vi "PH_Tektronix_7000.Evt Call Set Acquisition Configuration.vi"(0 "i ref in":refnum<vi>, 1 "Instance":string="N/A", 2 "Acquisition Configuration":T1={"Record Length"=0, "Timebase [s/div]"=10000.0, "Position [%]"=0.0, "Acquisition Type"=1, "Average Waveforms"=10, "Envelope Waveforms"=10, "WfmDB Samples"=16000, "Continuous?"=FALSE, "Delay [s]"=0.0, "Run?"=FALSE} {"Delay [s]" format="%#_12p"; "Acquisition Type" items=["Sample", "Peak Detect", "Hi Res", "Average", "Envelope", "WfmDB"]; "Timebase [s/div]" format="%#_12g"}, 5 "error in (no error)":errorcluster) -> (14 "i ref out":refnum<vi>, 19 "error out":errorcluster)   [LabVIEW 2014, in "PH_Tektronix_7000.lvlib"]
doc: "This VI calls sets a simple call."
uses:
  PH_Tektronix_7000.lvlib
  PH_Tektronix_7000.Acquisition Config.ctl
  CSCore/CSSystem/CoreLib/CoreLib.int 2 byte array.vi
  CSCore/CSSystem/CoreLib/CoreLib.double 2 byte array.vi
  CSCore/CSSystem/CoreLib/CoreLib.short 2 byte array.vi
  CSCore/CSSystem/CoreLib/CoreLib.lvlib
  CSCore/BaseProcess/BaseProcess.lvlib
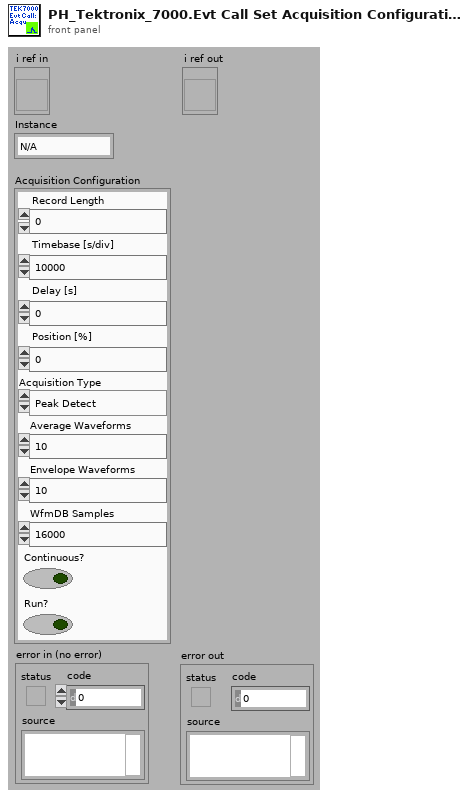
[diagram p1: front panel]
types:
  T1 = typedef "PH_Tektronix_7000.lvlib/PH_Tektronix_7000.Acquisition Config.ctl" = cluster{"Record Length":u32, "Timebase [s/div]":dbl, "Position [%]":dbl, "Acquisition Type":u16, "Average Waveforms":i32, "Envelope Waveforms":i32, "WfmDB Samples":i32, "Continuous?":bool, "Delay [s]":dbl, "Run?":bool}
  T2 = typedef "CoreDefs.rawDataType.ctl" = i8[]
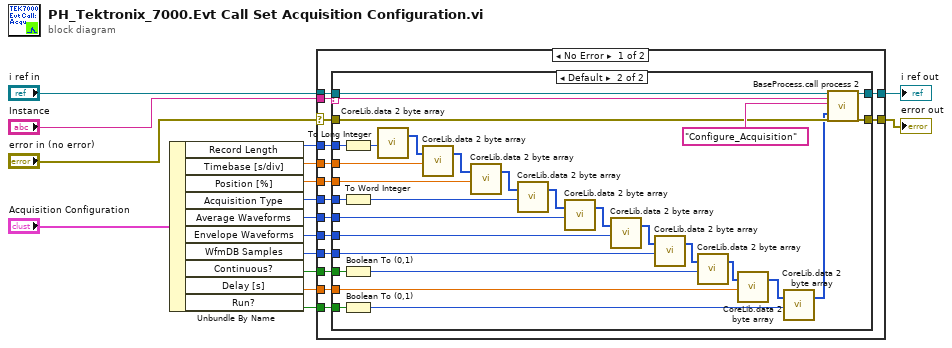
[diagram p0: block diagram]
diagram:
  n1 = Unbundle By Name("Acquisition Configuration") -> ("Record Length"=w10:u32, "Timebase [s/div]"=w9:dbl, "Position [%]"=w8:dbl, "Acquisition Type"=w7:u16, "Average Waveforms"=w6:i32, "Envelope Waveforms"=w4:i32, "WfmDB Samples"=w3:i32, "Continuous?"=w5:bool, "Delay [s]"=w2:dbl, "Run?"=w1:bool)
  n2 = case shown="No Error" "error in (no error)" {
    selector: "error in (no error)" -> [w27 w64]
    tunnel: [w31 w65] -> w16
    tunnel: [w30 w64] -> w15
    tunnel: "i ref in" -> [w29 w65]
    tunnel: w10 -> [w26 _]
    tunnel: "Instance" -> [w28 _]
    tunnel: w9 -> [w25 _]
    tunnel: w8 -> [w24 _]
    tunnel: w7 -> [w23 _]
    tunnel: w6 -> [w22 _]
    tunnel: w5 -> [w21 _]
    tunnel: w4 -> [w20 _]
    tunnel: w3 -> [w19 _]
    tunnel: w2 -> [w18 _]
    tunnel: w1 -> [w17 _]
    frame No Error {
      n3 = case shown="Default" w28 {
        selector: w28 -> [_ w58]
        tunnel: [w32 w62] -> w31
        tunnel: [w33 w61] -> w30
        tunnel: w29 -> [w32 w60]
        tunnel: w27 -> [w33 w59]
        tunnel: w26 -> [_ w57]
        tunnel: w25 -> [_ w48]
        tunnel: w24 -> [_ w55]
        tunnel: w23 -> [_ w53]
        tunnel: w22 -> [_ w46]
        tunnel: w21 -> [_ w50]
        tunnel: w20 -> [_ w44]
        tunnel: w19 -> [_ w42]
        tunnel: w18 -> [_ w39]
        tunnel: w17 -> [_ w38]
        frame "N/A" {
        }
        frame Default {
          n4 = To Long Integer(number=w57) -> (32bit integer=w49:i32)
          n5 = To Word Integer(number=w53) -> (16bit integer=w47:i16)
          n6 = Boolean To (0,1)(Boolean=w50) -> (0, 1=w52:i16)
          n7 = Boolean To (0,1)(Boolean=w38) -> (0, 1=w37:i16)
          n8 = call-poly "CoreLib.data 2 byte array.vi"("i32"=w49) -> ("byteArray out"=w56:T2)  [unwired: 18 in]
          n9 = call-poly "CoreLib.data 2 byte array.vi"("byteArray"=w56, "f64"=w48) -> ("byteArray out"=w54:T2)  [unwired: 17 in]
          n10 = call-poly "CoreLib.data 2 byte array.vi"("byteArray"=w54, "f64"=w55) -> ("byteArray out"=w51:T2)  [unwired: 17 in]
          n11 = call-poly "CoreLib.data 2 byte array.vi"("byteArray"=w51, "i16"=w47) -> ("byteArray out"=w45:T2)  [unwired: 17 in]
          n12 = call-poly "CoreLib.data 2 byte array.vi"("byteArray"=w45, "i32"=w46) -> ("byteArray out"=w43:T2)  [unwired: 17 in]
          n13 = call-poly "CoreLib.data 2 byte array.vi"("byteArray"=w43, "i32"=w44) -> ("byteArray out"=w41:T2)  [unwired: 17 in]
          n14 = call-poly "CoreLib.data 2 byte array.vi"("byteArray"=w41, "i32"=w42) -> ("byteArray out"=w34:T2)  [unwired: 17 in]
          n15 = call-poly "CoreLib.data 2 byte array.vi"("byteArray"=w34, "i16"=w52) -> ("byteArray out"=w40:T2)  [unwired: 17 in]
          n16 = call-poly "CoreLib.data 2 byte array.vi"("byteArray"=w40, "f64"=w39) -> ("byteArray out"=w36:T2)  [unwired: 17 in]
          n17 = call-poly "CoreLib.data 2 byte array.vi"("byteArray"=w36, "i16"=w37) -> ("byteArray out"=w35:T2)  [unwired: 17 in]
          n18 = call "BaseProcess.call process 2.vi"("i ref in"=w60, "Object"=w58, "Selector"="Configure_Acquisition", "Data"=w35, "error in (no error)"=w59) -> ("i ref out"=w62:refnum<vi>, "error out"=w61:errorcluster)  [unwired: 13 in]
        }
      }
    }
    frame Error {
    }
  }
  "i ref out" <- w16
  "error out" <- w15
